vi "Drive_AutoShift.vi"(7 "Max":dbl format="%#_13g", 8 "Right  Input":dbl, 9 "Left Input":dbl, 10 "Right RPM":dbl, 11 "Left RPM":dbl) -> (1 "Shifting":bool, 2 "Right Output":dbl, 3 "Left Output":dbl)   [LabVIEW 2016]
uses:
  <vilib>/Rock Robotics/WPI/Solenoid/WPI_SolenoidValue.ctl
  Robot Global Data.vi
panel:
  # "Used to be 1770, for some reason it is now 830."
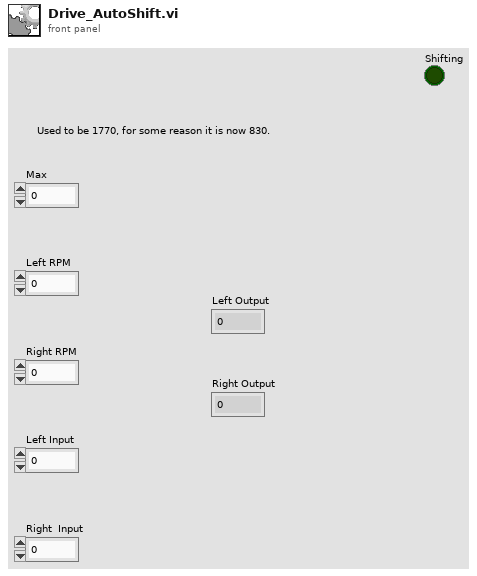
[diagram p1: front panel]
types:
  T1 = typedef "WPI_SolenoidValue.ctl" = enum16{"Off", "On", "Forward", "Reverse"}
  T2 = typedef "WPI_SolenoidDevRef.ctl" = cluster{"DevStatus":errorcluster, "Pneumatics Control Module":u8, "Forward Solenoid Channel":T3, "Reverse Solenoid Channel":T3}
  T3 = typedef "WPI_SolenoidChannel.ctl" = enum8{"Solenoid 0", "Solenoid 1", "Solenoid 2", "Solenoid 3", "Solenoid 4", "Solenoid 5", "Solenoid 6", "Solenoid 7", "Invalid"}
  T4 = cluster{"OutputMAX":dbl, "OutputMIN":dbl, "InputMAX":dbl, "InputMIN":dbl}
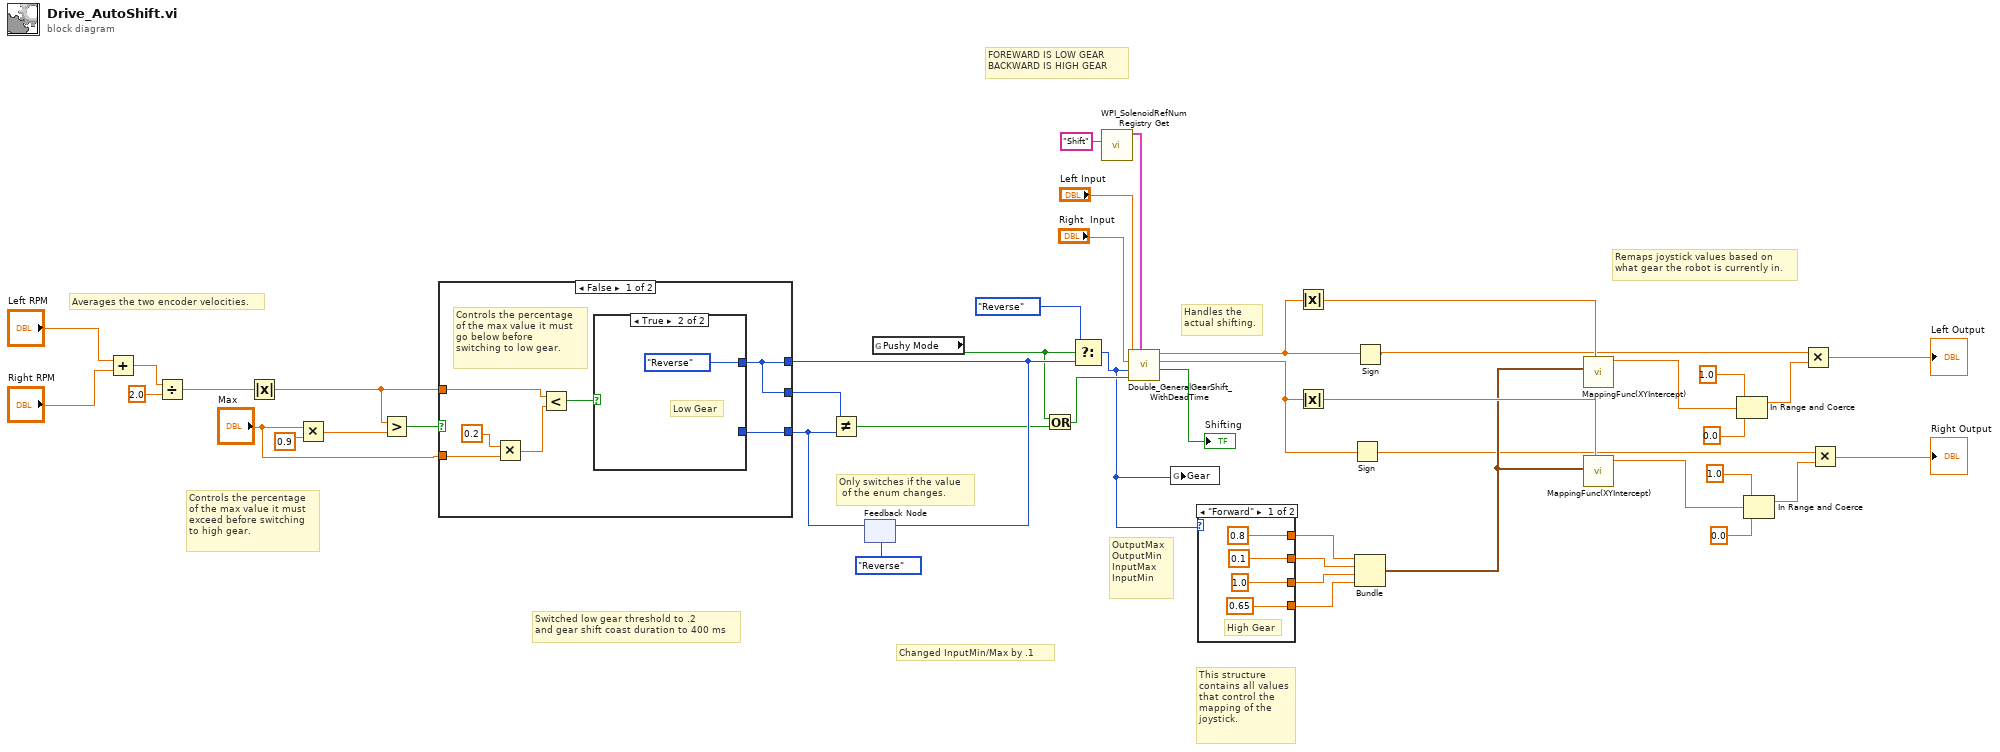
[diagram p0: block diagram]
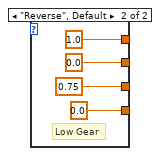
[diagram p2: hidden frame]
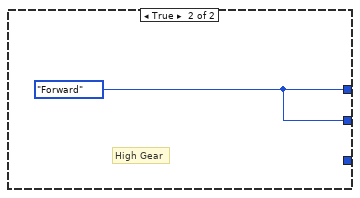
[diagram p4: hidden frame]
diagram:
  # "Switched low gear threshold to .2\nand gear shift coast duration to 400 ms"
  # "Changed InputMin/Max by .1"
  # "OutputMax\nOutputMin\nInputMax\nInputMin"
  # "This structure\ncontains all values\nthat control the\nmapping of the \njoystick."
  # "Remaps joystick values based on\nwhat gear the robot is currently in."
  # "Handles the\nactual shifting."
  # "FOREWARD IS LOW GEAR\nBACKWARD IS HIGH GEAR"
  # "Only switches if the value\n of the enum changes."
  # "Controls the percentage\nof the max value it must \nexceed before switching\nto high gear."
  # "Averages the two encoder velocities."
  n1 = Add(x="Left RPM", y="Right RPM") -> (x+y=w30:dbl)
  n2 = Divide(x=w30, y=2.0) -> (x/y=w6:dbl)
  n3 = Absolute Value(x=w6) -> (abs(x)=w5:dbl)
  n4 = Multiply(x="Max", y=0.9) -> (x*y=w44:dbl)
  n5 = Greater?(x=w5, y=w44) -> (0:w43:bool)
  n6 = feedback #1(WPI_SolenoidValue."Reverse" ("Shift Value")) -> (w41:T1)
  n7 = case shown="False" w43 {
    tunnel: [w48 w55] -> w20
    tunnel: [w48 w55] -> w42
    tunnel: "Max" -> [w51 _]
    tunnel: w41 -> [w47 _]
    tunnel: w5 -> [w46 _]
    frame False {
      # "Controls the percentage\nof the max value it must \ngo below before \nswitching to low gear."
      n8 = Multiply(x=0.2, y=w51) -> (x*y=w49:dbl)
      n9 = Less?(x=w46, y=w49) -> (x < y?=w52:bool)
      n10 = case shown="True" w52 {
        tunnel: [w53 WPI_SolenoidValue."Reverse" ("Shift Value")] -> w48
        tunnel: w47 -> [w53 _]
        frame False {
        }
        frame True {
          # "Low Gear"
        }
      }
    }
    frame True {
      w55 = WPI_SolenoidValue."Forward" ("Shift Value")
      # "High Gear"
    }
  }
  n11 = Not Equal?(x=w42, y=w41) -> (x != y?=w3:bool)
  n12 = feedback-in #1(w20) -> ()
  n13 = global read "Robot Global Data.vi" "Pushy Mode"() -> (w4:bool)
  n14 = Or(x=w4, y=w3) -> (x .or. y?=w2:bool)
  n15 = Select(t=WPI_SolenoidValue."Reverse", s=w4, f=w20) -> (s? t:f=w1:T1)
  n16 = call <vilib>:"WPI_SolenoidRefNum Registry Get.vi"("refnum name"="Shift") -> ("SolenoidDevRef"=w38:T2)  [unwired: 9 in, 1 out]
  n17 = call "Double_GeneralGearShift_WithDeadTime.vi"("ShifterRef"=w38, "Shift Control"=w2, "Shift Value"=w1, "Right"="Right  Input", "Left"="Left Input") -> ("Shifting"=→"Shifting":bool, "Right Output"=w14:dbl, "Left Output"=w12:dbl)  [unwired: 3 in, 1 out]
  n18 = global write "Robot Global Data.vi" "Gear"(w1) -> ()
  n19 = case shown="\"Forward\"" w1 {
    tunnel: [0.8 ("OutputMAX") 1.0 ("OutputMAX")] -> w17
    tunnel: [0.1 ("OutputMIN") 0.0 ("OutputMIN")] -> w16
    tunnel: [1.0 ("InputMAX") 0.75 ("InputMAX")] -> w18
    tunnel: [0.65 ("InputMIN") 0.0 ("InputMIN")] -> w19
    frame "Forward" {
      # "High Gear"
    }
    frame "Reverse", Default {
      # "Low Gear"
    }
  }
  n20 = Absolute Value(x=w12) -> (abs(x)=w35:dbl)
  n21 = Absolute Value(x=w14) -> (abs(x)=w25:dbl)
  n22 = Sign(1:w14) -> (0:w13:dbl)
  n23 = Sign(1:w12) -> (0:w11:dbl)
  n24 = Bundle("OutputMAX"=w17, "OutputMIN"=w16, "InputMAX"=w18, "InputMIN"=w19) -> (w15:T4)  [unwired: 1 in]
  n25 = call "MappingFunc(XYIntercept).vi"("Input"=w35, "Cluster"=w15) -> ("Output"=w34:dbl)  [unwired: 9 in]
  n26 = call "MappingFunc(XYIntercept).vi"("Input"=w25, "Cluster"=w15) -> ("Output"=w26:dbl)  [unwired: 9 in]
  n27 = In Range and Coerce(upper limit=1.0, x=w34, lower limit=0.0) -> (coerced(x)=w31:dbl)  [unwired: 1 out]
  n28 = In Range and Coerce(upper limit=1.0, x=w26, lower limit=0.0) -> (coerced(x)=w27:dbl)  [unwired: 1 out]
  n29 = Multiply(x=w11, y=w31) -> (x*y=→"Left Output":dbl)
  n30 = Multiply(x=w13, y=w27) -> (x*y=→"Right Output":dbl)
